vi "MathLoop.vi"(7 "CORE":refnum<queue>, 8 "error in (no error)":errorcluster, 9 "Solve notifier":refnum<notifier>, 10 "MATH":refnum<queue>, 11 "ACQ Data Queue":T1) -> (0 "error out":errorcluster)   [LabVIEW 2014, in "MathLoop.lvlib"]
doc: "Loop encargado de configurar, convertir, procesar y calcular las operaciones matemáticas que se apliquen en el programa principal."
uses:
  MathLoop.lvlib
  APIs/Message Queue/Message Cluster.ctl
  APIs/Data Queue/All Data Queues Cluster.ctl
  APIs/Data Queue/Acquisition Data 1 Sample Cluster.ctl
  APIs/Data Queue/Control Data Cluster.ctl
  APIs/Data Queue/Async Acquisition Data Cluster.ctl
  TypeDefs/NumericData.ctl
  TypeDefs/ParsedExpression.ctl
  TypeDefs/typeMed.ctl
  TypeDefs/Conf. Gral.ctl
  Solve/Aux&ResultSolve/ResultSolver.vi
  <vilib>/Analysis/baseanly.llb/Mean.vi
  <vilib>/Analysis/baseanly.llb/Mean (DBL).vi
  <vilib>/Analysis/2dsp.llb/FFT.vi
  <vilib>/Analysis/2dsp.llb/Real FFT.vi
  <vilib>/Analysis/2dsp.llb/Inverse FFT.vi
  <vilib>/Analysis/2dsp.llb/Inverse Complex FFT.vi
  Solve/Aux&ResultSolve/RPNSolver.vi
  TypeDefs/Globals.vi
  APIs/Message Queue/Enqueue Message (Single).vi
  APIs/Message Queue/WINFAS 2 Message Queue.lvlib
  APIs/Data Queue/WINFAS 2 Data Queue.lvlib
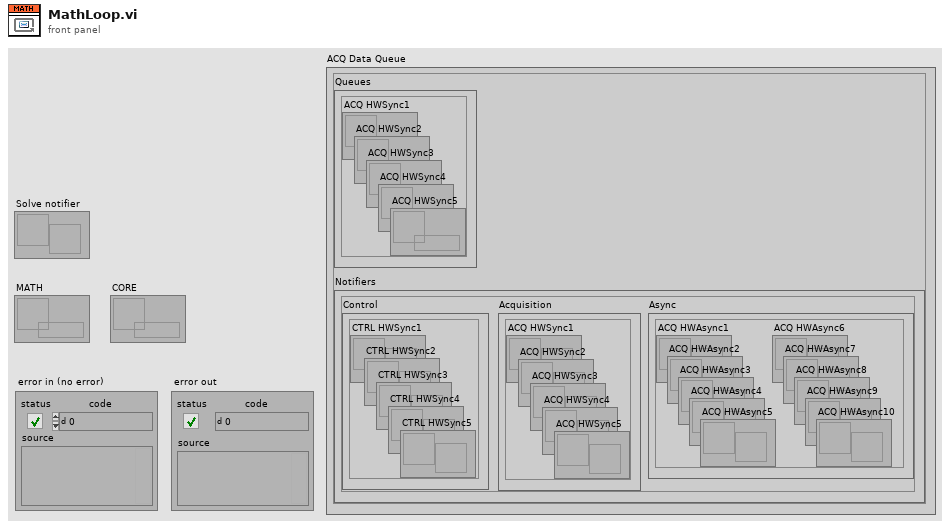
[diagram p1: front panel]
types:
  T1 = typedef "WINFAS 2 Data Queue.lvlib/All Data Queues Cluster.ctl" = cluster{"Queues":cluster{"ACQ HWSync1":refnum<queue>, "ACQ HWSync2":refnum<queue>, "ACQ HWSync3":refnum<queue>, "ACQ HWSync4":refnum<queue>, "ACQ HWSync5":refnum<queue>}, "Notifiers":cluster{"Control":cluster{"CTRL HWSync1":refnum<notifier>, "CTRL HWSync2":refnum<notifier>, "CTRL HWSync3":refnum<notifier>, "CTRL HWSync4":refnum<notifier>, "CTRL HWSync5":refnum<notifier>}, "Acquisition":cluster{"ACQ HWSync1":refnum<notifier>, "ACQ HWSync2":refnum<notifier>, "ACQ HWSync3":refnum<notifier>, "ACQ HWSync4":refnum<notifier>, "ACQ HWSync5":refnum<notifier>}, "Async":cluster{"ACQ HWAsync1":refnum<notifier>, "ACQ HWAsync2":refnum<notifier>, "ACQ HWAsync3":refnum<notifier>, "ACQ HWAsync4":refnum<notifier>, "ACQ HWAsync5":refnum<notifier>, "ACQ HWAsync6":refnum<notifier>, "ACQ HWAsync7":refnum<notifier>, "ACQ HWAsync8":refnum<notifier>, "ACQ HWAsync9":refnum<notifier>, "ACQ HWAsync10":refnum<notifier>}}}
  T2 = typedef "MathLoop.lvlib/ParsedExpression.ctl" = cluster{"RPN ":string[], "Constantes":sgl[], "Variables":string[], "Formula":string, "Tipo de Med":T3, "Med?":bool, "Descripción":string, "Nominal":sgl, "Tol Sup":sgl, "Pre TS":sgl, "Pre TI":sgl, "Tol Inf":sgl}
  T3 = typedef "MathLoop.lvlib/typeMed.ctl" = string
  T4 = typedef "MathLoop.lvlib/Conf. Gral.ctl" = cluster{"Engranometro":cluster{"Cant. Dientes x pieza":i32, "Nro. Dientes (Frp)":i32, "Armonicas":i32}}
  T5 = cluster{"Variable Data Out":cluster{"Kcte":sgl[], "Dcte":sgl[], "Aux":sgl[][], "Transductores":sgl[][]}, "Array":sgl[], T2[], "Array Med":sgl[][], "Conf. General":T4}
  T6 = typedef "MathLoop.lvlib/NumericData.ctl" = cluster{"Kcte":sgl[], "Dcte":sgl[], "Aux":sgl[][], "Transductores":sgl[][]}
  T7 = cluster{"ACQ HWSync1":refnum<queue>, "ACQ HWSync2":refnum<queue>, "ACQ HWSync3":refnum<queue>, "ACQ HWSync4":refnum<queue>, "ACQ HWSync5":refnum<queue>}
  T8 = cluster{"Kcte":sgl[], "Dcte":sgl[], "Aux":sgl[][], "Transductores":sgl[][]}
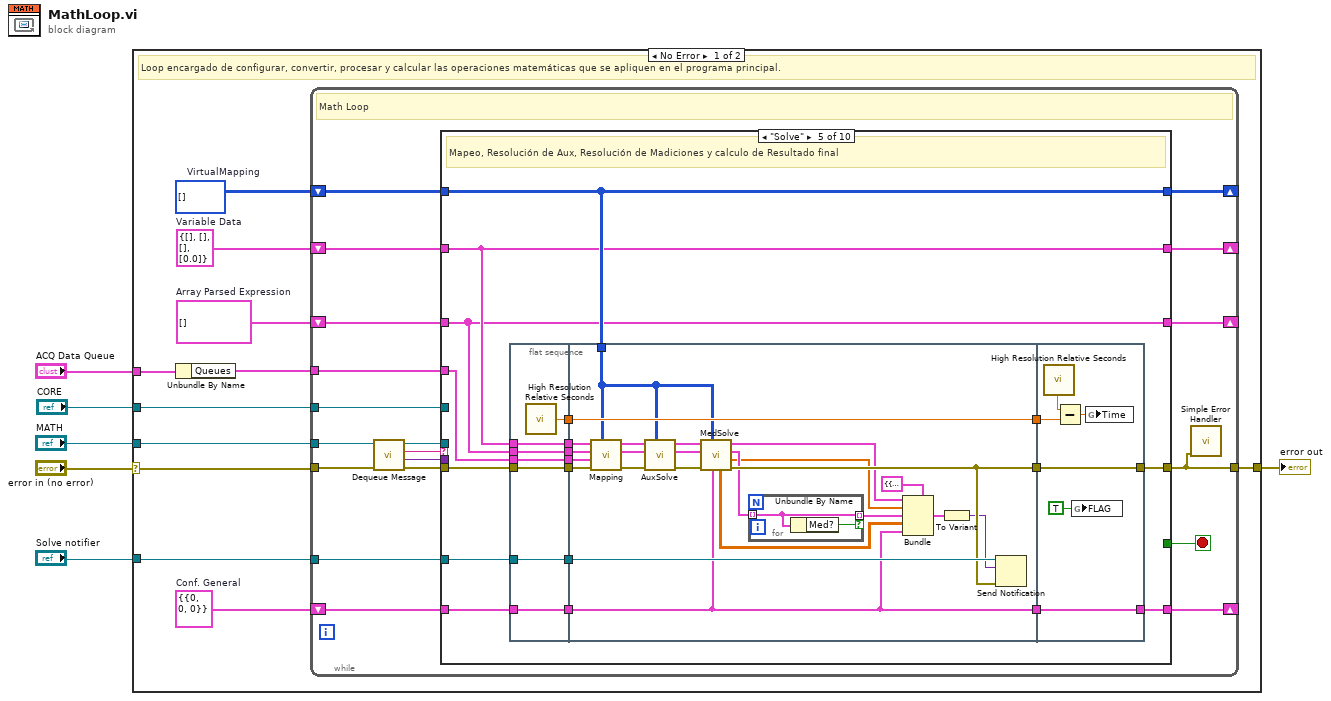
[diagram p0: block diagram]
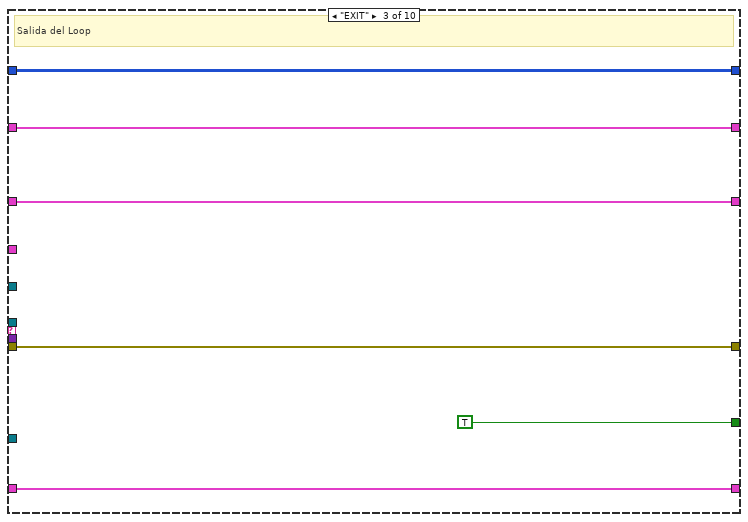
[diagram p4: hidden frame]
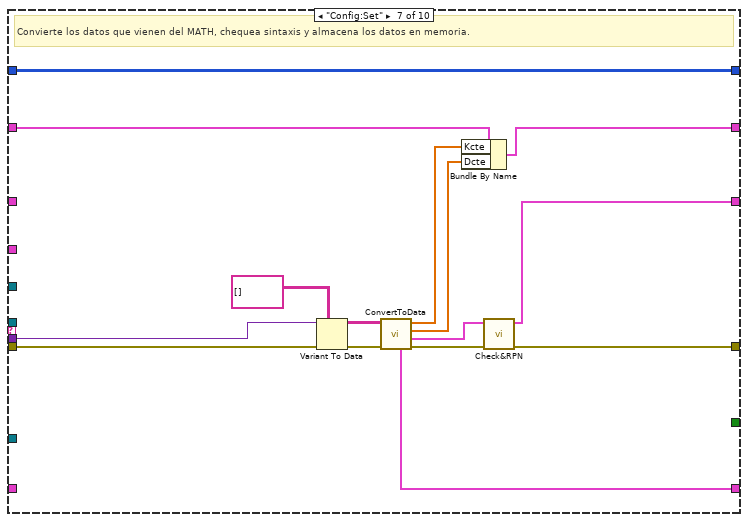
[diagram p7: hidden frame]
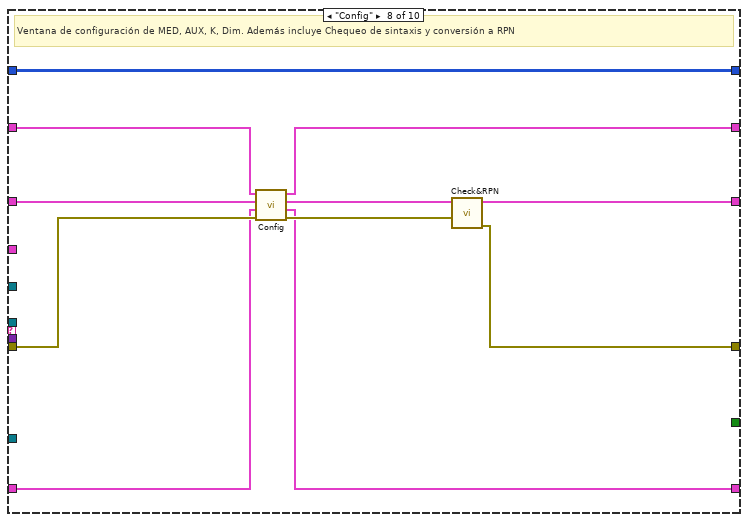
[diagram p8: hidden frame]
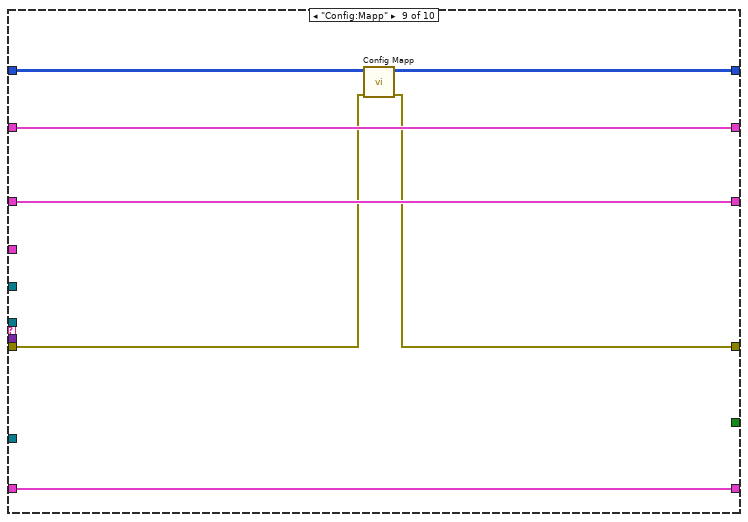
[diagram p9: hidden frame]
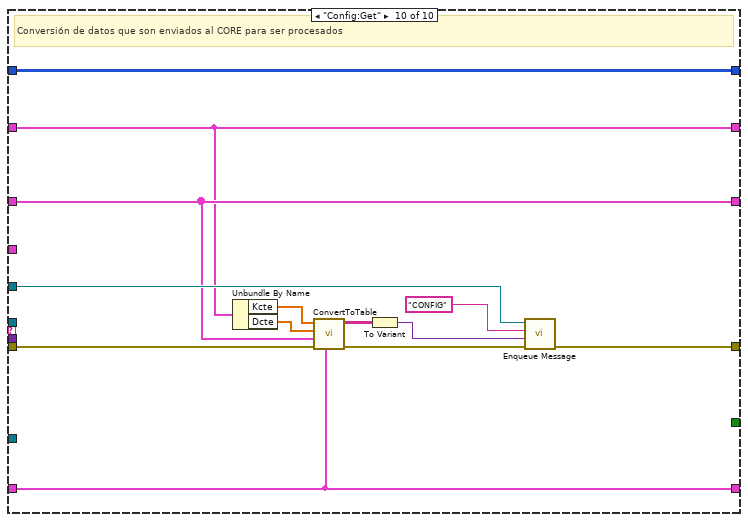
[diagram p10: hidden frame]
diagram:
  n1 = case shown="No Error" "error in (no error)" {
    selector: "error in (no error)" -> [w17 w166]
    tunnel: [w12 w166] -> w5
    tunnel: "MATH" -> [w13 _]
    tunnel: "ACQ Data Queue" -> [w16 _]
    tunnel: "Solve notifier" -> [w11 _]
    tunnel: "CORE" -> [w9 _]
    frame No Error {
      w7 = T4 {"Engranometro"={"Cant. Dientes x pieza"=0, "Nro. Dientes (Frp)"=0, "Armonicas"=0}}  # Conf. General
      w8 = u16[][] []  # VirtualMapping
      w10 = T2[] []  # Array Parsed Expression
      w14 = T6 {"Kcte"=[], "Dcte"=[], "Aux"=[], "Transductores"=[[0.0]]}  # Variable Data
      # "Loop encargado de configurar, convertir, procesar y calcular las operaciones matemáticas que se apliquen en el programa principal."
      n2 = Unbundle By Name(w16) -> ("Queues"=w15:T7)
      n3 = while {
        tunnel: w17 -> [w36]
        tunnel: [w20] -> w12
        tunnel: w13 -> [w25]
        tunnel: w15 -> [w31]
        shift-right: [w29] -> _
        shift-left: w10 -> [w28]
        shift-right: [w27] -> _
        shift-left: w14 -> [w26]
        tunnel: w11 -> [w24]
        shift-right: [w22] -> _
        shift-left: w8 -> [w23]
        tunnel: w9 -> [w21]
        shift-right: [w18] -> _
        shift-left: w7 -> [w19]
        stop <- w30 stop-if-true
        # "Math Loop"
        n4 = call "Dequeue Message.vi"("error in (no error)"=w36, "Message Queue"=w25) -> ("error out"=w32:errorcluster, "Message Data"=w33:variant, "Message"=w35:string, "dup Message Queue"=w34:refnum<queue>)  [unwired: 6 in]
        n5 = case shown="\"Solve\"" w35 {
          tunnel: w34 -> [_ _ _ _ _ _ _ _ _ _]
          tunnel: w33 -> [_ _ _ _ _ _ w133 _ _ _]
          tunnel: w32 -> [w41 w46 w52 w57 w76 w119 w132 w145 w147 w155]
          tunnel: [w41 w46 w52 w57 w73 w119 w121 w138 w146 w161] -> w20
          tunnel: w31 -> [_ _ _ _ w75 _ _ _ _ _]
          tunnel: [_ _ TRUE _ _ _ _ _ _ _] -> w30
          tunnel: w28 -> [w39 w44 w50 w55 w58 w117 _ w141 w151 w160]
          tunnel: [w39 w44 w50 w55 w58 w117 w123 w137 w151 w160] -> w29
          tunnel: [w40 w45 w49 w56 w59 w118 w128 w143 w152 w158] -> w27
          tunnel: w26 -> [w40 w45 w49 w56 w59 w118 w129 w142 w152 w158]
          tunnel: w24 -> [_ _ _ _ w74 _ _ _ _ _]
          tunnel: w23 -> [w38 w43 w48 w54 w65 w116 w134 w144 w149 w165]
          tunnel: [w38 w43 w48 w54 w65 w116 w134 w144 w148 w165] -> w22
          tunnel: w21 -> [_ _ _ _ _ _ _ _ _ w162]
          tunnel: [w37 w42 w47 w53 w63 w115 w120 w135 w150 w153] -> w18
          tunnel: w19 -> [w37 w42 w47 w53 w61 w115 _ w136 w150 w153]
          frame "----LOOP----" {
            # "Bloque que adminte futuras configuraciones al inicio."
          }
          frame Default {
          }
          frame "EXIT" {
            # "Salida del Loop"
          }
          frame "----ACTION----" {
            # "Bloque que adminte futuras configuraciones al inicio."
          }
          frame "Solve" {
            # "Mapeo, Resolución de Aux, Resolución de Madiciones y calculo de Resultado final"
            n6 = flat-sequence {
              tunnel: w74 -> [w83]
              tunnel: w75 -> [w80]
              tunnel: w59 -> [w82]
              tunnel: w58 -> [w81]
              tunnel: w76 -> [w79]
              tunnel: [w83] -> w70
              tunnel: [w82] -> w69
              tunnel: [w81] -> w68
              tunnel: [w80] -> w67
              tunnel: [w79] -> w66
              tunnel: [w78] -> w64
              tunnel: [w77] -> w62
              tunnel: w61 -> [w77]
              tunnel: [w105] -> w72
              tunnel: w70 -> [w106]
              tunnel: [w90] -> w71
              tunnel: w69 -> [w98]
              tunnel: w68 -> [w86]
              tunnel: w67 -> [w97]
              tunnel: w66 -> [w96]
              tunnel: w65 -> [w84]
              tunnel: w64 -> [w90]
              tunnel: w62 -> [w87]
              tunnel: [w87] -> w60
              tunnel: [w112] -> w73
              tunnel: w72 -> [w112]
              tunnel: w71 -> [w110]
              tunnel: [w109] -> w63
              tunnel: w60 -> [w109]
              frame #0 {
                n7 = call <vilib>:"High Resolution Relative Seconds.vi"() -> ("relative seconds"=w78:dbl)
              }
              frame #1 {
                n8 = call "Mapping.vi"("VirtualMapping"=w84, "error in (no error)"=w96, "Queues"=w97, "Array Parsed Expression"=w86, "Variable Data In"=w98) -> ("error out"=w94:errorcluster, "Array Parsed Expression Out"=w85:T2[], "Variable Data Out"=w95:T8)  [unwired: 4 in]
                n9 = call "AuxSolve.vi"("Variable Data in"=w95, "Array Parsed Expression in"=w85, "error in (no error)"=w94, "VirtualMapping"=w84) -> ("Variable Data Out"=w91:T8, "Array Parsed Expression Out"=w92:T2[], "error out"=w93:errorcluster)  [unwired: 4 in]
                n10 = call "MedSolve.vi"("Conf. Gral."=w87, "VirtualMapping"=w84, "error in (no error)"=w93, "Array Parsed Expression in"=w92, "Variable Data in"=w91) -> ("error out"=w105:errorcluster, "Array"=w89:sgl[], "Array Parsed Expression Out"=w104:T2[], "Variable Data Out"=w100:T8, "Array Med"=w99:sgl[][])  [unwired: 2 in]
                n11 = for {
                  tunnel: w104 -> [w108] mode=indexing
                  tunnel: [w108] -> w101 mode=indexing if=w107
                  n12 = Unbundle By Name(w108) -> ("Med?"=w107:bool)
                }
                n13 = Bundle(cluster=T5 {"Variable Data Out"={"Kcte"=[], "Dcte"=[], "Aux"=[], "Transductores"=[]}, "Array"=[], [], "Array Med"=[], "Conf. General"={"Engranometro"={"Cant. Dientes x pieza"=0, "Nro. Dientes (Frp)"=0, "Armonicas"=0}}} ("output cluster"), "Variable Data Out"=w100, "Array"=w89, w101, "Array Med"=w99, "Conf. General"=w87) -> (w103:T5)
                n14 = To Variant(anything=w103) -> (Variant=w102:variant)
                n15 = Send Notification(notification=w102, notifier=w106, error in (no error)=w105) -> ()  [unwired: 2 out]
              }
              frame #2 {
                n16 = call <vilib>:"High Resolution Relative Seconds.vi"() -> ("relative seconds"=w114:dbl)
                n17 = Subtract(x=w114, y=w110) -> (x-y=w113:dbl)
                n18 = global write "Globals.vi" "FLAG"(TRUE ("FLAG")) -> ()
                n19 = global write "Globals.vi" "Time"(w113) -> ()
              }
            }
          }
          frame "----UTILITY----" {
            # "Bloque que adminte futuras configuraciones al inicio."
          }
          frame "Config:Set" {
            # "Convierte los datos que vienen del MATH, chequea sintaxis y almacena los datos en memoria."
            n20 = Variant To Data(error in=w132, type=string[][] [], Variant=w133) -> (data=w131:string[][], error out=w125:errorcluster)
            n21 = call "ConvertToData.vi"("error in (no error)"=w125, "Mediciones"=w131) -> ("error out"=w122:errorcluster, "Array Parsed Expression Out"=w124:T2[], "Dcte"=w126:sgl[], "Kcte"=w127:sgl[], "Conf. Gral."=w120:T4)  [unwired: 5 in]
            n22 = Bundle By Name(cluster=w129, "Kcte"=w127, "Dcte"=w126) -> (w128:T6)
            n23 = call "Check&RPN.vi"("error in (no error)"=w122, "Array Parsed Expression"=w124) -> ("error out"=w121:errorcluster, "Array Parsed Expression"=w123:T2[])  [unwired: 8 in]
          }
          frame "Config" {
            # "Ventana de configuración de MED, AUX, K, Dim. Además incluye Chequeo de sintaxis y conversión a RPN"
            n24 = call "Config.vi"("error in (no error)"=w145, "Conf. Gral."=w136, "Array Parsed Expression"=w141, "Variable Data In"=w142) -> ("error out"=w139:errorcluster, "Conf. Gral. Out"=w135:T4, "Array Parsed Expression Out"=w140:T2[], "Variable Data Out"=w143:T6)  [unwired: 4 in]
            n25 = call "Check&RPN.vi"("error in (no error)"=w139, "Array Parsed Expression"=w140) -> ("error out"=w138:errorcluster, "Array Parsed Expression"=w137:T2[])  [unwired: 8 in]
          }
          frame "Config:Mapp" {
            n26 = call "Config Mapp.vi"("error in (no error)"=w147, "VirtualMapping"=w149) -> ("error out"=w146:errorcluster, "VirtualMapping"=w148:u16[][])  [unwired: 8 in]
          }
          frame "Config:Get" {
            # "Conversión de datos que son enviados al CORE para ser procesados"
            n27 = Unbundle By Name(w158) -> ("Kcte"=w157:sgl[], "Dcte"=w156:sgl[])
            n28 = call "ConvertToTable.vi"("Conf. Gral."=w153, "error in (no error)"=w155, "Array Parsed Expression In"=w160, "Dcte"=w156, "Kcte"=w157) -> ("error out"=w154:errorcluster, "Mediciones"=w159:string[][])  [unwired: 5 in]
            n29 = To Variant(anything=w159) -> (Variant=w164:variant)
            n30 = call-poly "Enqueue Message.vi"("error in (no error)"=w154, "Message Data"=w164, "Message"="CONFIG", "Message Queue"=w162) -> ("error out"=w161:errorcluster)  [unwired: 6 in, 1 out]
          }
        }
        n31 = call <vilib>:"Simple Error Handler.vi"("error in (no error)"=w20) -> ()  [unwired: 4 in, 5 out]
      }
    }
    frame Error {
    }
  }
  "error out" <- w5
